vi "disconnect.vi"(8 "error in (no error)":errorcluster, 11 "SpectrographClientCommunicator in":refnum<class "SpectrographClientCommunicator.lvclass">) -> (0 "error out":errorcluster, 3 "SpectrographClientCommunicator out":refnum<class "SpectrographClientCommunicator.lvclass">)   [LabVIEW 2016, in "SpectrographClientCommunicator.lvclass"]
uses:
  SpectrographClientCommunicator.lvclass
  ts_labview_tcp/TCPClient/TCPClient.lvclass
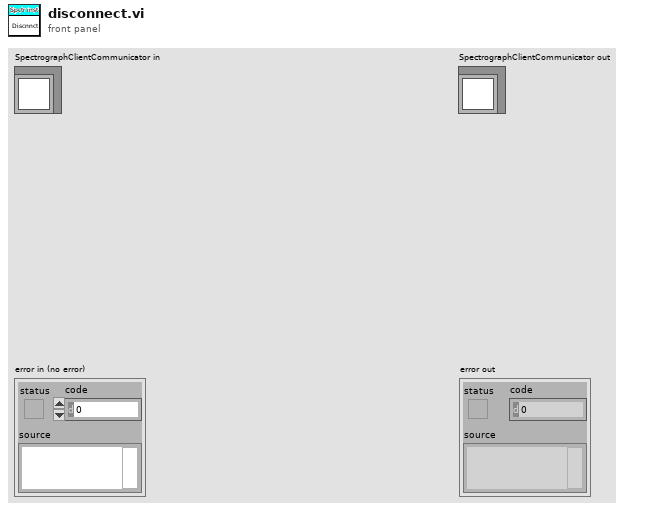
[diagram p1: front panel]
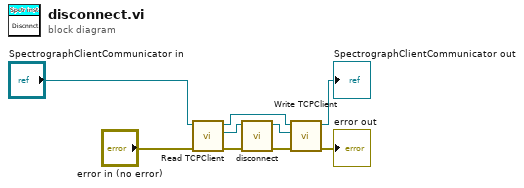
[diagram p0: block diagram]
diagram:
  n1 = call-dynamic "Read TCPClient.vi"("error in (no error)"="error in (no error)", "SpectrographClientCommunicator in"="SpectrographClientCommunicator in") -> ("error out"=w6:errorcluster, "TCPClient"=w9:refnum<class "TCPClient.lvclass">, "SpectrographClientCommunicator out"=w8:refnum<class "SpectrographClientCommunicator.lvclass">)  [unwired: 7 in]
  n2 = call-dynamic "disconnect.vi"("error in (no error)"=w6, "TCPClient in"=w9) -> ("error out"=w5:errorcluster, "TCPClient out"=w7:refnum<class "TCPClient.lvclass">)  [unwired: 8 in]
  n3 = call-dynamic "Write TCPClient.vi"("error in (no error)"=w5, "TCPClient"=w7, "SpectrographClientCommunicator in"=w8) -> ("error out"=→"error out":errorcluster, "SpectrographClientCommunicator out"=→"SpectrographClientCommunicator out":refnum<class "SpectrographClientCommunicator.lvclass">)  [unwired: 7 in]
